vi "MoveFromBallPlacementInterferenceSkill.vi"(4 "AdjustPositionInBallPlacement":bool, 6 "Ballposition(x,y)":dbl[](array[numeric]), 7 "projectionOfQInBallPlacementLine":dbl[](array[numeric]) format="%#_13g", 8 "error in (no error)":errorcluster, 9 "Game in":refnum<class "Game.lvclass">, 10 "Robot in":refnum<class "Robot.lvclass">, 11 "MoveFromBallPlacementInterferenceSkill in":refnum<class "MoveFromBallPlacementInterferenceSkill.lvclass">) -> (0 "error out":errorcluster, 2 "Robot out":refnum<class "Robot.lvclass">, 3 "MoveFromBallPlacementInterferenceSkill out":refnum<class "MoveFromBallPlacementInterferenceSkill.lvclass">)   [LabVIEW 2020, in "MoveFromBallPlacementInterferenceSkill.lvclass"]
uses:
  MoveFromBallPlacementInterferenceSkill.lvclass
  Game_class/Game.lvclass
  Robot_class/Robot.lvclass
  C:/Users/anton/Desktop/RoboIME/IC/SSL_AI/Object_class/Object.lvclass
  Object_class/Object.lvclass/Object.ctl
  Game_class/Game.lvclass/Game.ctl
  Robot_class/Robot.lvclass/Robot.ctl
  <vilib>/Analysis/coordinate.llb/2D Cartesian Coordinate Rotation (Scalar).vi
  <vilib>/Analysis/baseanly.llb/Unit Vector (DBL).vi
  <vilib>/Analysis/baseanly.llb/Real Dot Product.vi
  Game_class/Read Referee.vi
  Game_class/Read BallRef.vi
  Game_class/Read NewParameters.vi
  Game_class/Read FieldRef.vi
  Game_class/Read Utilities.lvclass.vi
  Object_class/Read x.vi
  Object_class/Read y.vi
  Robot_class/Write dest_x.vi
  Robot_class/Write dest_y.vi
  Field_class/Field.lvclass
  Utilities_class/Utilities.lvclass
  Referee_class/Referee.lvclass
  Ball_class/Ball.lvclass
  <vilib>/Analysis/NI_AALPro.lvlib
  <vilib>/Analysis/NI_AALBase.lvlib
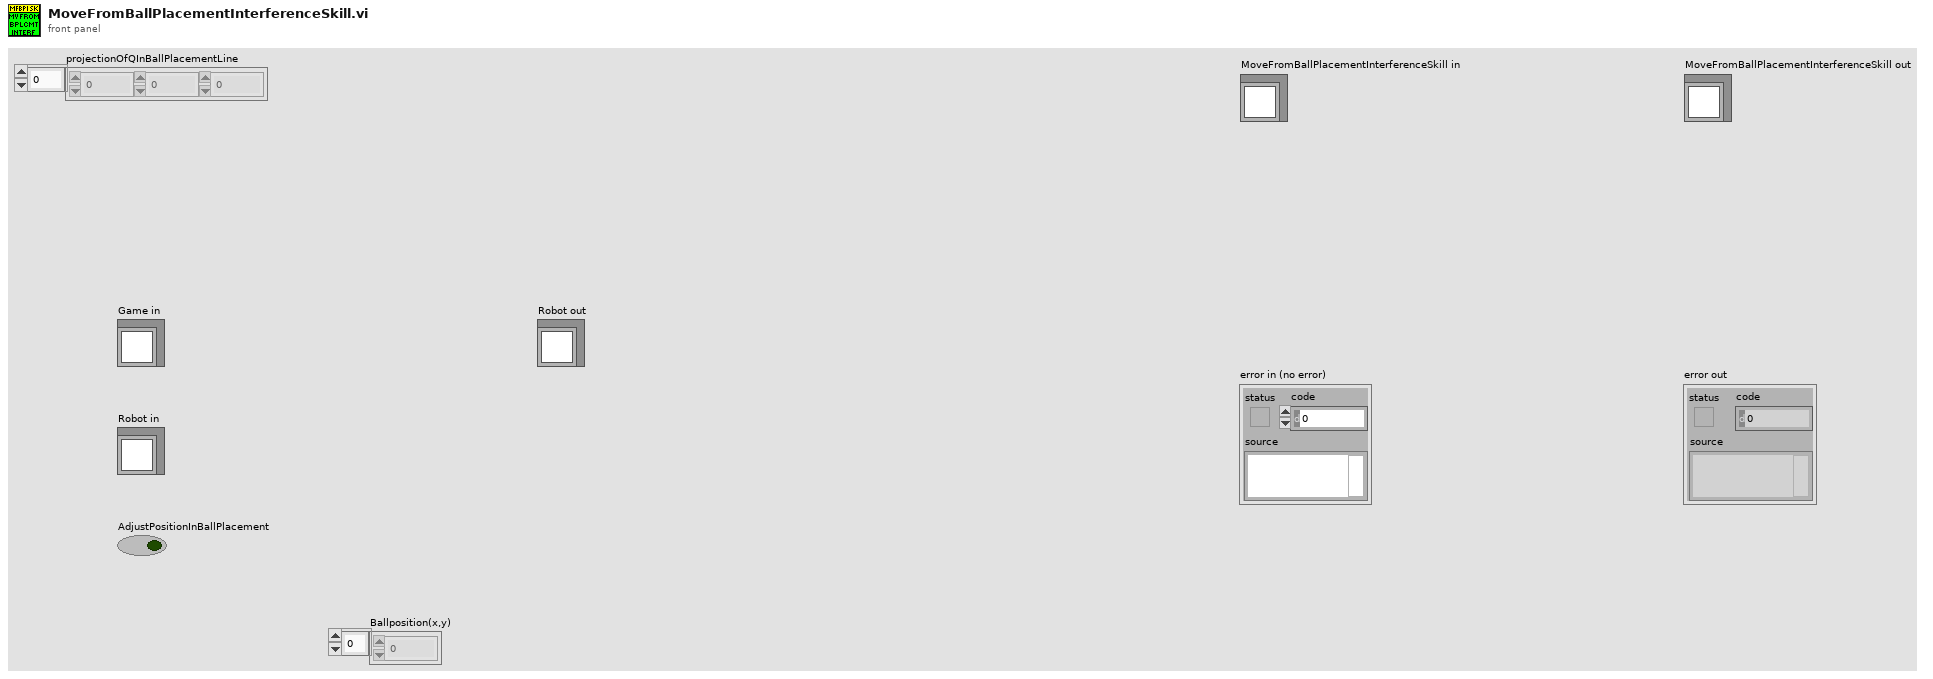
[diagram p1: front panel]
types:
  T1 = typedef "NewParameters.ctl" = cluster{"PenaltyDistance":dbl, "DistanceAttackerToBackBall":dbl, "Division":enum16{"Div B", "Div A"}, "DistanceToAvoidyEnemyRobot":dbl, "BallPlacementDistance":dbl, "DisatanceBehindBallToStealBall":dbl, "MaxDistanceToPositionKickoff":dbl, "BlockEnemyTarget":bool, "MaxStopVAng":dbl, "DistanceMarkerToEnemy":dbl, "IgnoreDribblerContact":bool, "DistanceToBeginEnemyPosession":dbl, "GoToBallWhenEnemyNotMoving":bool, "EnemyDistanceToReduceVelocity":dbl, "TurnOnEnemyDistanceToReduceVelocity":bool, "EnemyDistanceToShootOutBall":dbl, "DefenseKickBall":bool, "MoreKickToGoal? (0-0.3)":dbl, "ChipKickInEnemyField":bool, "ShootOutRobotId":dbl, "FieldLenghtDenominatorInShootOut":dbl, "AdjustPositionInBallPlacement":bool, "PowerGodPass":dbl, "VelocityAbortEnemyPos":dbl, "MaxDistToBeginPass":dbl, "MinDistToBeginPass":dbl, "VelocityInDirects":dbl, "BadDribblerIDs":i32[], "NewKickToDistanceAroundBall":dbl, "PowerAvoidColisionMarker":dbl, "DistanceToAvoidColisionMarker":dbl, "AvoidBallKick":dbl, "DistanceTryKick":dbl, "SuicideKickDIstance":dbl, "FirstKickAtck":bool, "AdjustFirstKickDistance":dbl, "FirstKickDefense":bool, "AvoidAimLessKick":dbl, "DistanceToAvoidyEnemyShootRobot ":dbl, "NumberOfMarkers":dbl, "PotField":bool, "PIDLateral":bool, "MinDistanceFirstKickX":dbl, "MinDistanceFirstKickY":dbl, "FractionOfDistToTouchGround\nAfterChipKick":dbl, "FractionOfKickxWhen\nComposedWithKickz":dbl, "Style":T2, "MoveInTurnState":bool, "DistFromEnemyToConsider\nMoveInTurnState":dbl}
  T2 = typedef "Style.ctl" = enum16{"Insanity", "Offensive", "Defensive"}
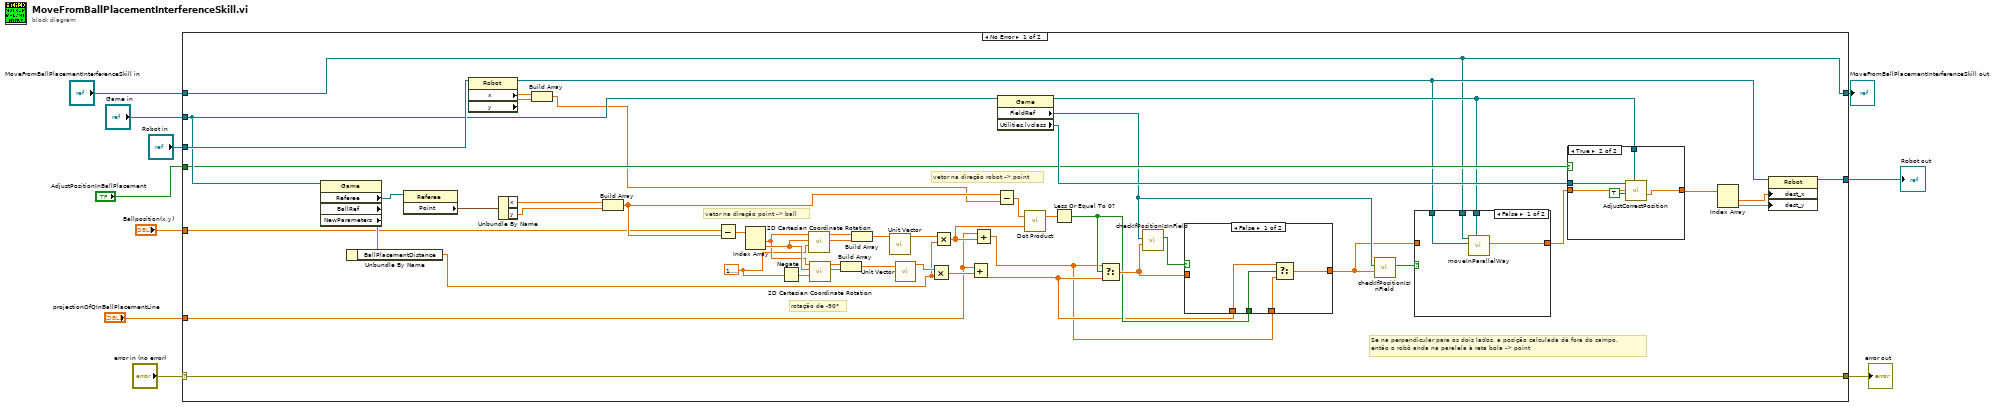
[diagram p0: block diagram]
diagram:
  n1 = case shown="No Error" "error in (no error)" {
    selector: "error in (no error)" -> [w60 w78]
    tunnel: [w60 w78] -> w9
    tunnel: [w11 w77] -> w7
    tunnel: "MoveFromBallPlacementInterferenceSkill in" -> [w11 w77]
    tunnel: "Robot in" -> [w28 _]
    tunnel: "Ballposition(x,y)" -> [w27 _]
    tunnel: "Game in" -> [w26 _]
    tunnel: "AdjustPositionInBallPlacement" -> [w25 _]
    tunnel: [w23 _] -> w2
    tunnel: "projectionOfQInBallPlacementLine" -> [w18 _]
    frame No Error {
      w37 = 1.5707963267948966
      # "Se na perpendicular para os dois lados, a posição calculada dá fora do campo,\nentão o robô anda na paralela à reta bola -> point"
      # "rotação de -90°"
      # "vetor na direção robot -> point"
      # "vetor na direção point -> ball"
      n2 = property class="Game" props=["Referee", "BallRef", "NewParameters"](reference=w26) -> ("Referee"=w29:refnum<class "Referee.lvclass">, "NewParameters"=w58:T1)  [unwired: 1 in, 3 out]
      n3 = Unbundle By Name(w58) -> ("BallPlacementDistance"=w24:dbl)
      n4 = property class="Referee"(reference=w29) -> ("Point"=w30:cluster{"x":sgl, "y":sgl})  [unwired: 1 in, 2 out]
      n5 = property class="Robot"(reference=w28) -> (reference out=w12:refnum<class "Robot.lvclass">, "x"=w33:dbl, "y"=w34:dbl)  [unwired: 1 in, 1 out]
      n6 = Unbundle By Name(w30) -> ("x"=w31:sgl, "y"=w32:sgl)
      n7 = Build Array(w33, w34) -> (w19:dbl[])
      n8 = Build Array(w31, w32) -> (w35:sgl[])
      n9 = Subtract(x=w27, y=w35) -> (x-y=w48:dbl[])
      n10 = Index Array(array=w48) -> (element #1=w38:dbl, element #2=w39:dbl)  [unwired: 2 in]
      n11 = Negate(x=w37) -> (-x=w36:dbl)
      n12 = call-poly <vilib>:"2D Cartesian Coordinate Rotation.vi"("theta"=w37, "y"=w39, "x"=w38) -> ("y out"=w41:dbl, "x out"=w40:dbl)  [unwired: 6 in, 1 out]
      n13 = call-poly <vilib>:"2D Cartesian Coordinate Rotation.vi"("theta"=w36, "y"=w39, "x"=w38) -> ("y out"=w43:dbl, "x out"=w42:dbl)  [unwired: 6 in, 1 out]
      n14 = Build Array(w42, w43) -> (w45:dbl[])
      n15 = Build Array(w40, w41) -> (w44:dbl[])
      n16 = call-poly <vilib>:"Unit Vector.vi"("Input Vector"=w44) -> ("Unit Vector"=w46:dbl[])  [unwired: 8 in, 2 out]
      n17 = call-poly <vilib>:"Unit Vector.vi"("Input Vector"=w45) -> ("Unit Vector"=w47:dbl[])  [unwired: 8 in, 2 out]
      n18 = Multiply(x=w47, y=w24) -> (x*y=w49:dbl[])
      n19 = Multiply(x=w46, y=w24) -> (x*y=w52:dbl[])
      n20 = Add(x=w18, y=w49) -> (x+y=w55:dbl[])
      n21 = Add(x=w18, y=w52) -> (x+y=w54:dbl[])
      n22 = Subtract(x=w35, y=w19) -> (x-y=w50:dbl[])
      n23 = property class="Game"(reference=w26) -> (reference out=w13:refnum<class "Game.lvclass">, "FieldRef"=w17:refnum<class "Field.lvclass">, "Utilities.lvclass"=w59:refnum<class "Utilities.lvclass">)  [unwired: 1 in, 1 out]
      n24 = call-poly <vilib>:"Dot Product.vi"("Y Vector"=w52, "X Vector"=w50) -> ("X * Y"=w51:dbl)  [unwired: 1 out]
      n25 = Less Or Equal To 0?(x=w51) -> (x <= 0?=w56:bool)
      n26 = Select(t=w54, s=w56, f=w55) -> (s? t:f=w57:dbl[])
      n27 = call "checkIfPositionIsInField.vi"("Position"=w57, "FieldRef"=w17) -> ("Position Is In Field?"=w53:bool)  [unwired: 5 in, 4 out]
      n28 = case shown="False" w53 {
        tunnel: w57 -> [_ w76]
        tunnel: [w72 w76] -> w14
        tunnel: w54 -> [w73 _]
        tunnel: w55 -> [w74 _]
        tunnel: w56 -> [w75 _]
        frame False {
          n29 = Select(t=w74, s=w75, f=w73) -> (s? t:f=w72:dbl[])
        }
        frame True {
        }
      }
      n30 = call "checkIfPositionIsInField.vi"("Position"=w14, "FieldRef"=w17) -> ("Position Is In Field?"=w16:bool)  [unwired: 5 in, 4 out]
      n31 = case shown="False" w16 {
        tunnel: [w64 w65] -> w15
        tunnel: w14 -> [_ w65]
        tunnel: w13 -> [w63 _]
        tunnel: w12 -> [w62 _]
        tunnel: w11 -> [w61 _]
        frame False {
          n32 = call "moveInParallelWay.vi"("Game"=w63, "Robot"=w62, "MoveFromBallPlacementInterferenceSkill in"=w61) -> ("finalPositionToGo"=w64:dbl[])  [unwired: 6 in, 2 out]
        }
        frame True {
        }
      }
      n33 = case shown="True" w25 {
        tunnel: w13 -> [_ w71]
        tunnel: w15 -> [w66 w70]
        tunnel: [w66 w69] -> w22
        tunnel: w59 -> [_ w68]
        frame False {
        }
        frame True {
          n34 = call "AdjustCorrectPosition.vi"("Game"=w71, "IsShoot?"=TRUE, "Position"=w70, "Utilities in"=w68) -> ("AdjustPosition"=w69:dbl[])  [unwired: 5 in, 2 out]
        }
      }
      n35 = Index Array(array=w22) -> (element #1=w21:dbl, element #2=w20:dbl)  [unwired: 2 in]
      n36 = property class="Robot"(reference=w12, "dest_x"=w21, "dest_y"=w20) -> (reference out=w23:refnum<class "Robot.lvclass">)  [unwired: 1 in, 1 out]
    }
    frame Error {
    }
  }
  "error out" <- w9
  "MoveFromBallPlacementInterferenceSkill out" <- w7
  "Robot out" <- w2
